vi "Project And Illuminate Triangle.vi"(4 "Alpha":dbl, 5 "Light Direction":T1={"x"=0.0, "y"=0.0, "z"=-1.0}, 6 "Diffuse Colour":u32(colorbox)=12517256, 7 "Screen Dimensions":T7, 8 "Name":string, 9 "Normal":T1, 10 "Projection Matrix":sgl[][](array[numeric]), 11 "Triangle in":T2={"Vertex 1"={"Position"={"x"=0.0, "y"=0.0, "z"=0.0}, "UV"={"u"=0.0, "v"=0.0}, "Colour"=12517256}, "Vertex 2"={"Position"={"x"=0.0, "y"=0.0, "z"=0.0}, "UV"={"u"=0.0, "v"=0.0}, "Colour"=12517256}, "Vertex 3"={"Position"={"x"=0.0, "y"=0.0, "z"=0.0}, "UV"={"u"=0.0, "v"=0.0}, "Colour"=12517256}, "Alpha"=0.0, "Alpha Blending Enabled"=FALSE, "Colour"=0, "Material"={"Diffuse Colour"=0, "Texture"={"Pixels"=refnum, "Size"={"Width"=0, "Height"=0}}}} {"Vertex 3"."UV"."v" min=0 max=1 step=0.1; "Vertex 3"."UV"."u" min=0 max=1 step=0.1; "Vertex 2"."UV"."v" min=0 max=1 step=0.1; "Vertex 2"."UV"."u" min=0 max=1 step=0.1; "Vertex 1"."UV"."v" min=0 max=1 step=0.1; "Vertex 1"."UV"."u" min=0 max=1 step=0.1}) -> (3 "Triangle out":T2={"Vertex 1"={"Position"={"x"=0.0, "y"=0.0, "z"=0.0}, "UV"={"u"=0.0, "v"=0.0}, "Colour"=12517256}, "Vertex 2"={"Position"={"x"=0.0, "y"=0.0, "z"=0.0}, "UV"={"u"=0.0, "v"=0.0}, "Colour"=12517256}, "Vertex 3"={"Position"={"x"=0.0, "y"=0.0, "z"=0.0}, "UV"={"u"=0.0, "v"=0.0}, "Colour"=12517256}, "Alpha"=12517256.0, "Alpha Blending Enabled"=FALSE, "Colour"=0, "Material"={"Diffuse Colour"=0, "Texture"={"Pixels"=refnum, "Size"={"Width"=0, "Height"=0}}}} {"Vertex 3"."UV"."v" min=0 max=1 step=0.1; "Vertex 3"."UV"."u" min=0 max=1 step=0.1; "Vertex 2"."UV"."v" min=0 max=1 step=0.1; "Vertex 2"."UV"."u" min=0 max=1 step=0.1; "Vertex 1"."UV"."v" min=0 max=1 step=0.1; "Vertex 1"."UV"."u" min=0 max=1 step=0.1})   [LabVIEW 2020, in "3D (FPGA).lvlib"]
uses:
  3D (FPGA).lvlib
  Vector 3D.ctl
  Raster/Rectangle Dimensions.ctl
  Raster/Raster (FPGA).lvlib
  Raster/UV.ctl
  Vertex.ctl
  Triangle.ctl
  Raster/Texture.ctl
  Material.ctl
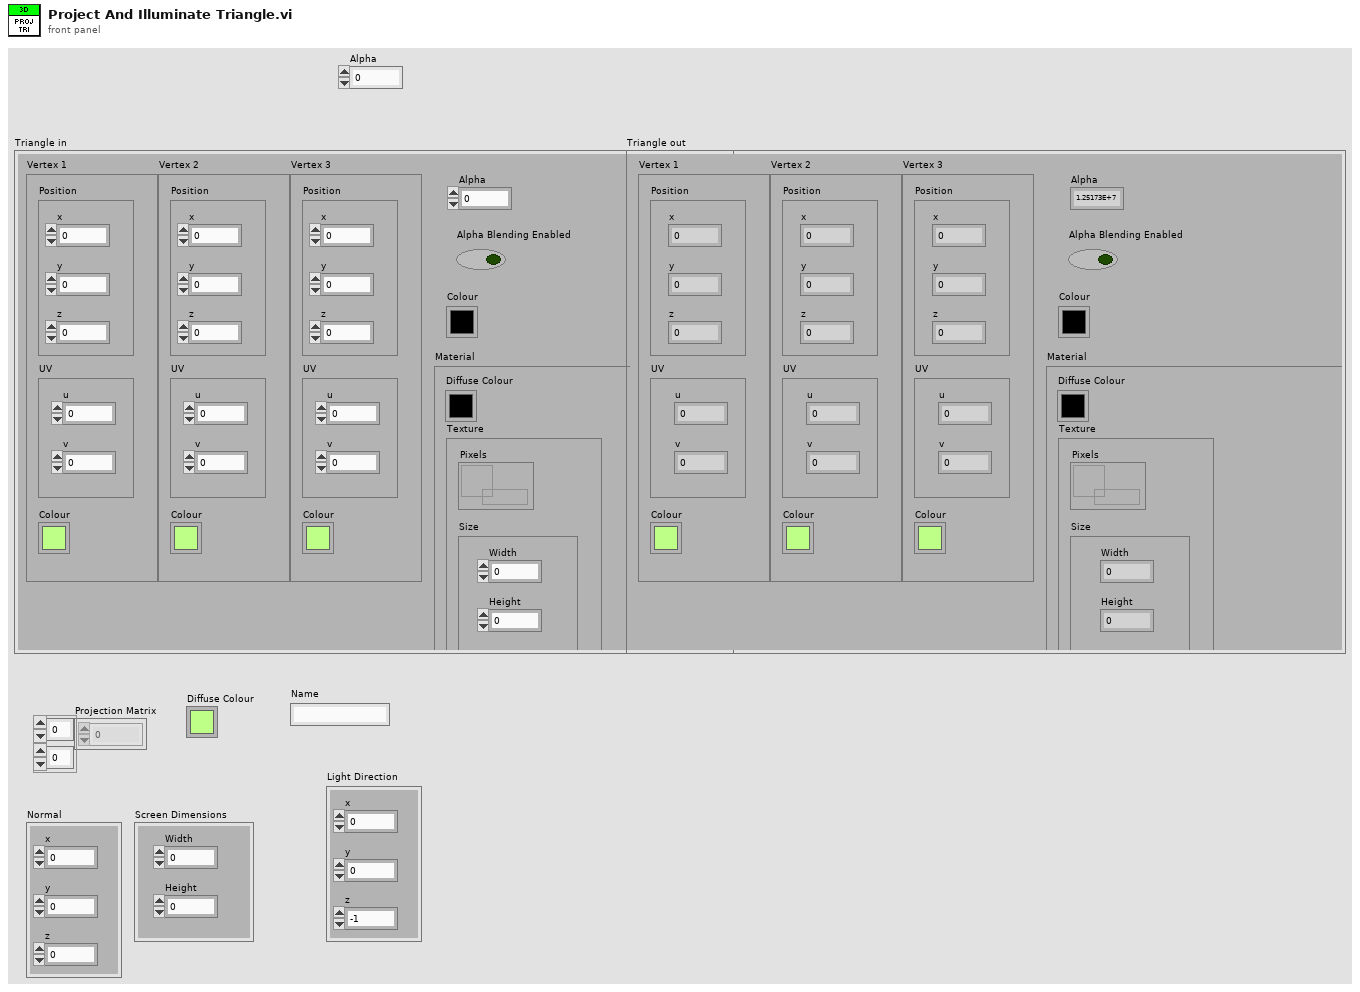
[diagram p1: front panel]
types:
  T1 = typedef "3D (FPGA).lvlib/Vector 3D.ctl" = cluster{"x":sgl, "y":sgl, "z":sgl}
  T2 = typedef "3D (FPGA).lvlib/Triangle.ctl" = cluster{"Vertex 1":T3, "Vertex 2":T3, "Vertex 3":T3, "Alpha":dbl, "Alpha Blending Enabled":bool, "Colour":u32, "Material":T5}
  T3 = typedef "3D (FPGA).lvlib/Vertex.ctl" = cluster{"Position":T1, "UV":T4, "Colour":u32}
  T4 = typedef "Raster (FPGA).lvlib/UV.ctl" = cluster{"u":sgl, "v":sgl}
  T5 = typedef "3D (FPGA).lvlib/Material.ctl" = cluster{"Diffuse Colour":u32, "Texture":T6}
  T6 = typedef "Raster (FPGA).lvlib/Texture.ctl" = cluster{"Pixels":refnum<data-value>, "Size":T7}
  T7 = typedef "Raster (FPGA).lvlib/Rectangle Dimensions.ctl" = cluster{"Width":u32, "Height":u32}
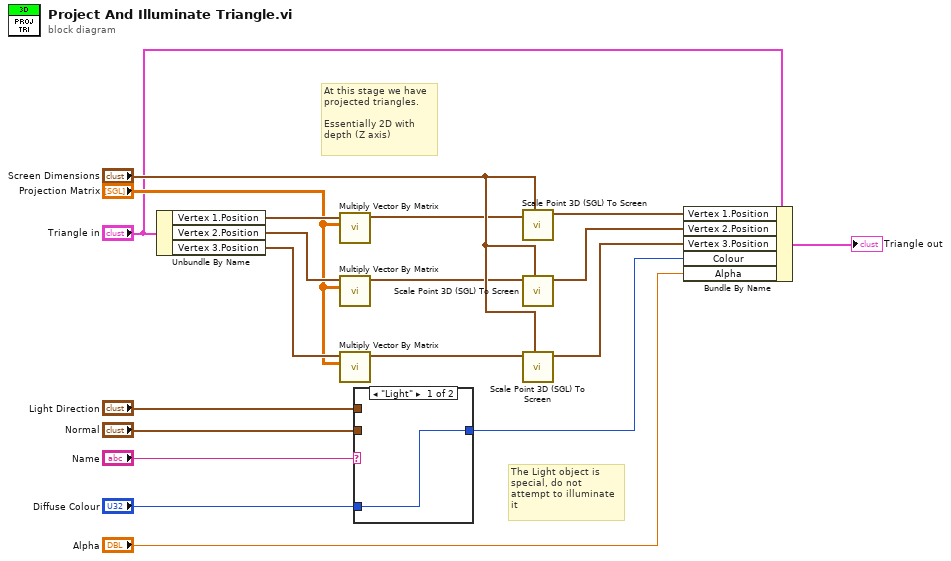
[diagram p0: block diagram]
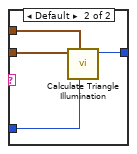
[diagram p2: hidden frame]
diagram:
  # "The Light object is special, do not attempt to illuminate it"
  # "At this stage we have projected triangles.\n\nEssentially 2D with depth (Z axis)"
  n1 = Unbundle By Name("Triangle in") -> ("Vertex 1.Position"=w17:T1, "Vertex 2.Position"=w18:T1, "Vertex 3.Position"=w19:T1)
  n2 = call "Multiply Vector By Matrix.vi"("Matrix in"="Projection Matrix", "Vector 3D in"=w17) -> ("Vector 3D out"=w11:T1)  [unwired: 9 in]
  n3 = call "Multiply Vector By Matrix.vi"("Matrix in"="Projection Matrix", "Vector 3D in"=w18) -> ("Vector 3D out"=w9:T1)  [unwired: 9 in]
  n4 = call "Multiply Vector By Matrix.vi"("Matrix in"="Projection Matrix", "Vector 3D in"=w19) -> ("Vector 3D out"=w10:T1)  [unwired: 9 in]
  n5 = case shown="\"Light\"" "Name" {
    tunnel: "Normal" -> [_ w24]
    tunnel: [w20 w23] -> w13
    tunnel: "Light Direction" -> [_ w22]
    tunnel: "Diffuse Colour" -> [w20 w21]
    frame "Light" {
    }
    frame Default {
      n6 = call "Calculate Triangle Illumination.vi"("Fill Colour"=w21, "Light Direction"=w22, "Triangle Normal"=w24) -> ("Fill Colour Actual"=w23:u32)  [unwired: 8 in]
    }
  }
  n7 = call "Scale Point 3D (SGL) To Screen.vi"("Screen Dimensions"="Screen Dimensions", "Point In"=w11) -> ("Point Out"=w6:T1)  [unwired: 9 in]
  n8 = call "Scale Point 3D (SGL) To Screen.vi"("Screen Dimensions"="Screen Dimensions", "Point In"=w9) -> ("Point Out"=w7:T1)  [unwired: 9 in]
  n9 = call "Scale Point 3D (SGL) To Screen.vi"("Screen Dimensions"="Screen Dimensions", "Point In"=w10) -> ("Point Out"=w8:T1)  [unwired: 9 in]
  n10 = Bundle By Name(cluster="Triangle in", "Vertex 1.Position"=w6, "Vertex 2.Position"=w7, "Vertex 3.Position"=w8, "Colour"=w13, "Alpha"="Alpha") -> (→"Triangle out":T2)
